vi "Ridge.vi"(8 "error in":errorcluster) -> (0 "error out":errorcluster, 3 "out":refnum<class "Ridge.lvclass">)   [LabVIEW 2020]
doc: "Linear least squares with l2 regularization.\n\n Minimizes the objective function::\n\n ||y - Xw||^2_2 + alpha * ||w||^2_2\n\n This model solves a regression model where the loss function is\n the linear least squares function and regularization is given by\n the l2-norm. Also known as Ridge Regression or Tikhonov regularization.\n This estimator has built-in support for multi-variate regression\n (i.e., when y is a 2d-array of shape (n_samples, n_targets)).\n\n Read more in the :ref:`User Guide <ridge_regression>`.\n\n Parameters\n ----------\n alpha : {float, ndarray of shape (n_targets,)}, default=1.0\n Regularization strength; must be a positive float. Regularization\n improves the conditioning of the problem and reduces the variance of\n the estimates. Larger values specify stronger regularization.\n Alpha corresponds to ``1 / (2C)`` in other linear models such as\n :class:`~sklearn.linear_model.LogisticRegression` or\n :class:`~sklearn.svm.LinearSVC`. If an array is passed, penalties are\n assumed to be specific to the targets. Hence they must correspond in\n number.\n\n fit_intercept : bool, default=True\n Whether to fit the intercept for this model. If set\n to false, no intercept will be used in calculations\n (i.e. ``X`` and ``y`` are expected to be centered).\n\n normalize : bool, default=False\n This parameter is ignored when ``fit_intercept`` is set to False.\n If True, the regressors X will be normalized before regression by\n subtracting the mean and dividing by the l2-norm.\n If you wish to standardize, please use\n :class:`~sklearn.preprocessing.StandardScaler` before calling ``fit``\n on an estimator with ``normalize=False``.\n\n copy_X : bool, default=True\n If True, X will be copied; else, it may be overwritten.\n\n max_iter : int, default=None\n Maximum number of iterations for conjugate gradient solver.\n For 'sparse_cg' and 'lsqr' solvers, the default value is determined\n by scipy.sparse.linalg. For 'sag' solver, the default value is 1000.\n\n tol : float, default=1e-3\n Precision of the solution.\n\n solver : {'auto', 'svd', 'cholesky', 'lsqr', 'sparse_cg', 'sag', 'saga'}, default='auto'\n Solver to use in the computational routines:\n\n - 'auto' chooses the solver automatically based on the type of data.\n\n - 'svd' uses a Singular Value Decomposition of X to compute the Ridge\n coefficients. More stable for singular matrices than 'cholesky'.\n\n - 'cholesky' uses the standard scipy.linalg.solve function to\n obtain a closed-form solution.\n\n - 'sparse_cg' uses the conjugate gradient solver as found in\n scipy.sparse.linalg.cg. As an iterative algorithm, this solver is\n more appropriate than 'cholesky' for large-scale data\n (possibility to set `tol` and `max_iter`).\n\n - 'lsqr' uses the dedicated regularized least-squares routine\n scipy.sparse.linalg.lsqr. It is the fastest and uses an iterative\n procedure.\n\n - 'sag' uses a Stochastic Average Gradient descent, and 'saga' uses\n its improved, unbiased version named SAGA. Both methods also use an\n iterative procedure, and are often faster than other solvers when\n both n_samples and n_features are large. Note that 'sag' and\n 'saga' fast convergence is only guaranteed on features with\n approximately the same scale. You can preprocess the data with a\n scaler from sklearn.preprocessing.\n\n All last five solvers support both dense and sparse data. However, only\n 'sag' and 'sparse_cg' supports sparse input when `fit_intercept` is\n True.\n\n .. versionadded:: 0.17\n Stochastic Average Gradient descent solver.\n .. versionadded:: 0.19\n SAGA solver.\n\n random_state : int, RandomState instance, default=None\n Used when ``solver`` == 'sag' or 'saga' to shuffle the data.\n See :term:`Glossary <random_state>` for details.\n\n .. versionadded:: 0.17\n `random_state` to support Stochastic Average Gradient.\n\n Attributes\n ----------\n coef_ : ndarray of shape (n_features,) or (n_targets, n_features)\n Weight vector(s).\n\n intercept_ : float or ndarray of shape (n_targets,)\n Independent term in decision function. Set to 0.0 if\n ``fit_intercept = False``.\n\n n_iter_ : None or ndarray of shape (n_targets,)\n Actual number of iterations for each target. Available only for\n sag and lsqr solvers. Other solvers will return None.\n\n .. versionadded:: 0.17\n\n See Also\n --------\n RidgeClassifier : Ridge classifier.\n RidgeCV : Ridge regression with built-in cross validation.\n :class:`~sklearn.kernel_ridge.KernelRidge` : Kernel ridge regression\n combines ridge regression with the kernel trick.\n\n \nAvailable methods:\nGet Attributes\nGet Params\nSet Params"
uses:
  Ridge.lvclass
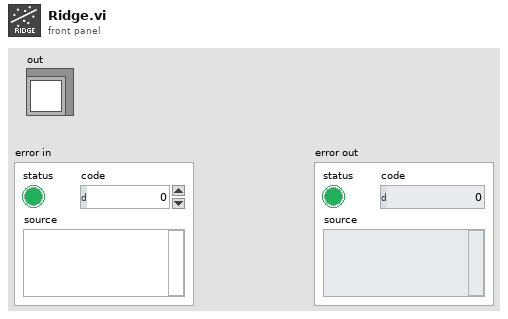
[diagram p1: front panel]
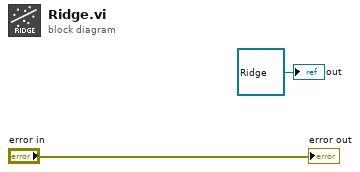
[diagram p0: block diagram]
diagram:
  "out" <- refnum<class "Ridge.lvclass"> refnum ("model")
  "error out" <- "error in"
